vi "armff_arm_sim_init.vi"() -> (3 "SingleJointArmSim":T1 {"GearBox"."Jr_KgM2" format="%13.5p"; "GearBox"."L_H" format="%13.5p"; "GearBox"."Kt_NMPerAmp" format="%13.5p"; "GearBox"."KvINV_RadPerSecPerVolt" format="%13.5p"; "GearBox"."R_Ohms" format="%13.5p"; "GearBox"."FreeSpeed_RadPerSec" format="%13.5p"; "GearBox"."FreeCurrent_Amps" format="%13.5p"; "GearBox"."StallCurrent_Amps" format="%13.5p"; "GearBox"."StallTorque_NM" format="%13.5p"; "GearBox"."nominalVoltage_Volts" format="%13.5p"})   [LabVIEW 2019]
uses:
  <vilib>/Rock Robotics/WPI/ThirdParty/JAS_Junk/TrajLib/Trajectory_Library.lvlib
  <vilib>/Analysis/Matrix/Datatypes/RealMatrix.ctl
  <vilib>/Analysis/Matrix/NI_Matrix.lvlib
  <vilib>/Rock Robotics/WPI/ThirdParty/JAS_Junk/TrajLib/TypeDef/LINEAR_SYSTEM.ctl
  <vilib>/Rock Robotics/WPI/ThirdParty/JAS_Junk/TrajLib/TypeDef/LINEAR_SYSTEM_SIM.ctl
  <vilib>/Rock Robotics/WPI/ThirdParty/JAS_Junk/TrajLib/TypeDef/DCMOTOR.CTL
  <vilib>/Rock Robotics/WPI/ThirdParty/JAS_Junk/TrajLib/TypeDef/SINGLE_JOINT_ARM_SIM.ctl
panel:
  # "<States, 1>"
  # "<Outputs, 1>"
  # "<Inputs, 1>"
  # "<Outputs, 1>"
  # "<States,States>"
  # "<States,Inputs>"
  # "<Outputs,States>"
  # "<Outputs,Inputs>"
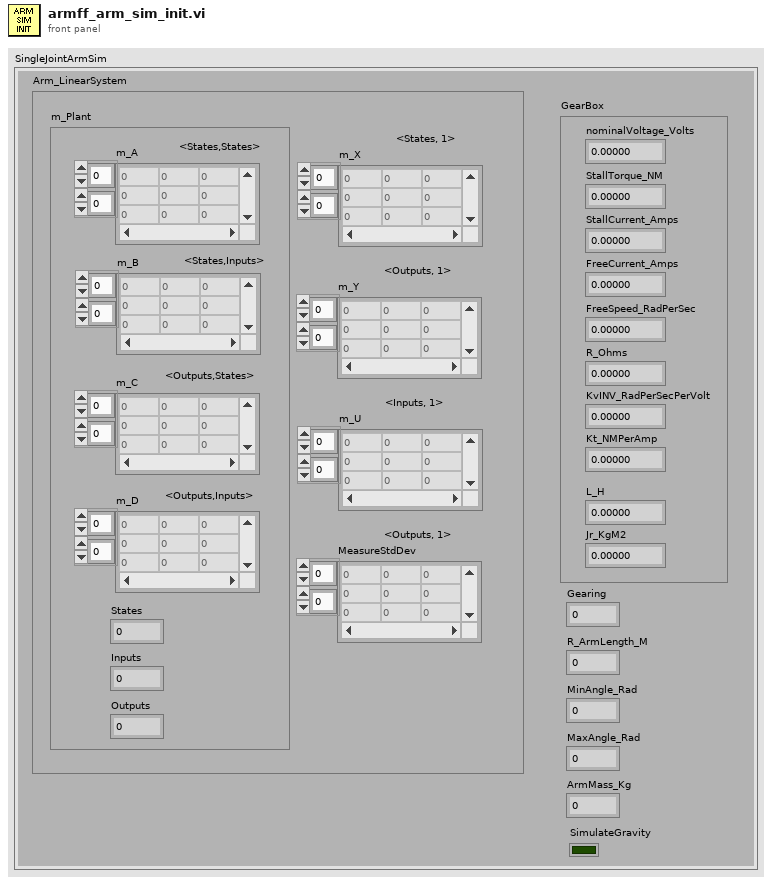
[diagram p1: front panel]
types:
  T1 = typedef "Trajectory_Library.lvlib/SINGLE_JOINT_ARM_SIM.ctl" = cluster{"Arm_LinearSystem":T2, "GearBox":T5, "Gearing":dbl, "R_ArmLength_M":dbl, "MinAngle_Rad":dbl, "MaxAngle_Rad":dbl, "ArmMass_Kg":dbl, "SimulateGravity":bool}
  T2 = typedef "Trajectory_Library.lvlib/LINEAR_SYSTEM_SIM.ctl" = cluster{"m_Plant":T3, "m_X":T4, "m_Y":T4, "m_U":T4, "MeasureStdDev":T4}
  T3 = typedef "Trajectory_Library.lvlib/LINEAR_SYSTEM.ctl" = cluster{"m_A":T4, "m_B":T4, "m_C":T4, "m_D":T4, "States":i32, "Inputs":i32, "Outputs":i32}
  T4 = typedef "NI_Matrix.lvlib/RealMatrix.ctl" = dbl[][]
  T5 = typedef "Trajectory_Library.lvlib/DCMOTOR.CTL" = cluster{"nominalVoltage_Volts":dbl, "StallTorque_NM":dbl, "StallCurrent_Amps":dbl, "FreeCurrent_Amps":dbl, "FreeSpeed_RadPerSec":dbl, "R_Ohms":dbl, "KvINV_RadPerSecPerVolt":dbl, "Kt_NMPerAmp":dbl, "L_H":dbl, "Jr_KgM2":dbl}
  T6 = typedef "Trajectory_Library.lvlib/KALMAN_FILTER.ctl" = cluster{"m_K":T4, "m_xHat":T4, "States":i32, "Outputs":i32, "m_Plant":T3}
  T7 = typedef "Trajectory_Library.lvlib/LINEAR_QUADRATIC_REGULATOR.ctl" = cluster{"m_r":T4, "m_U":T4, "m_K":T4, "States":i32, "Inputs":i32}
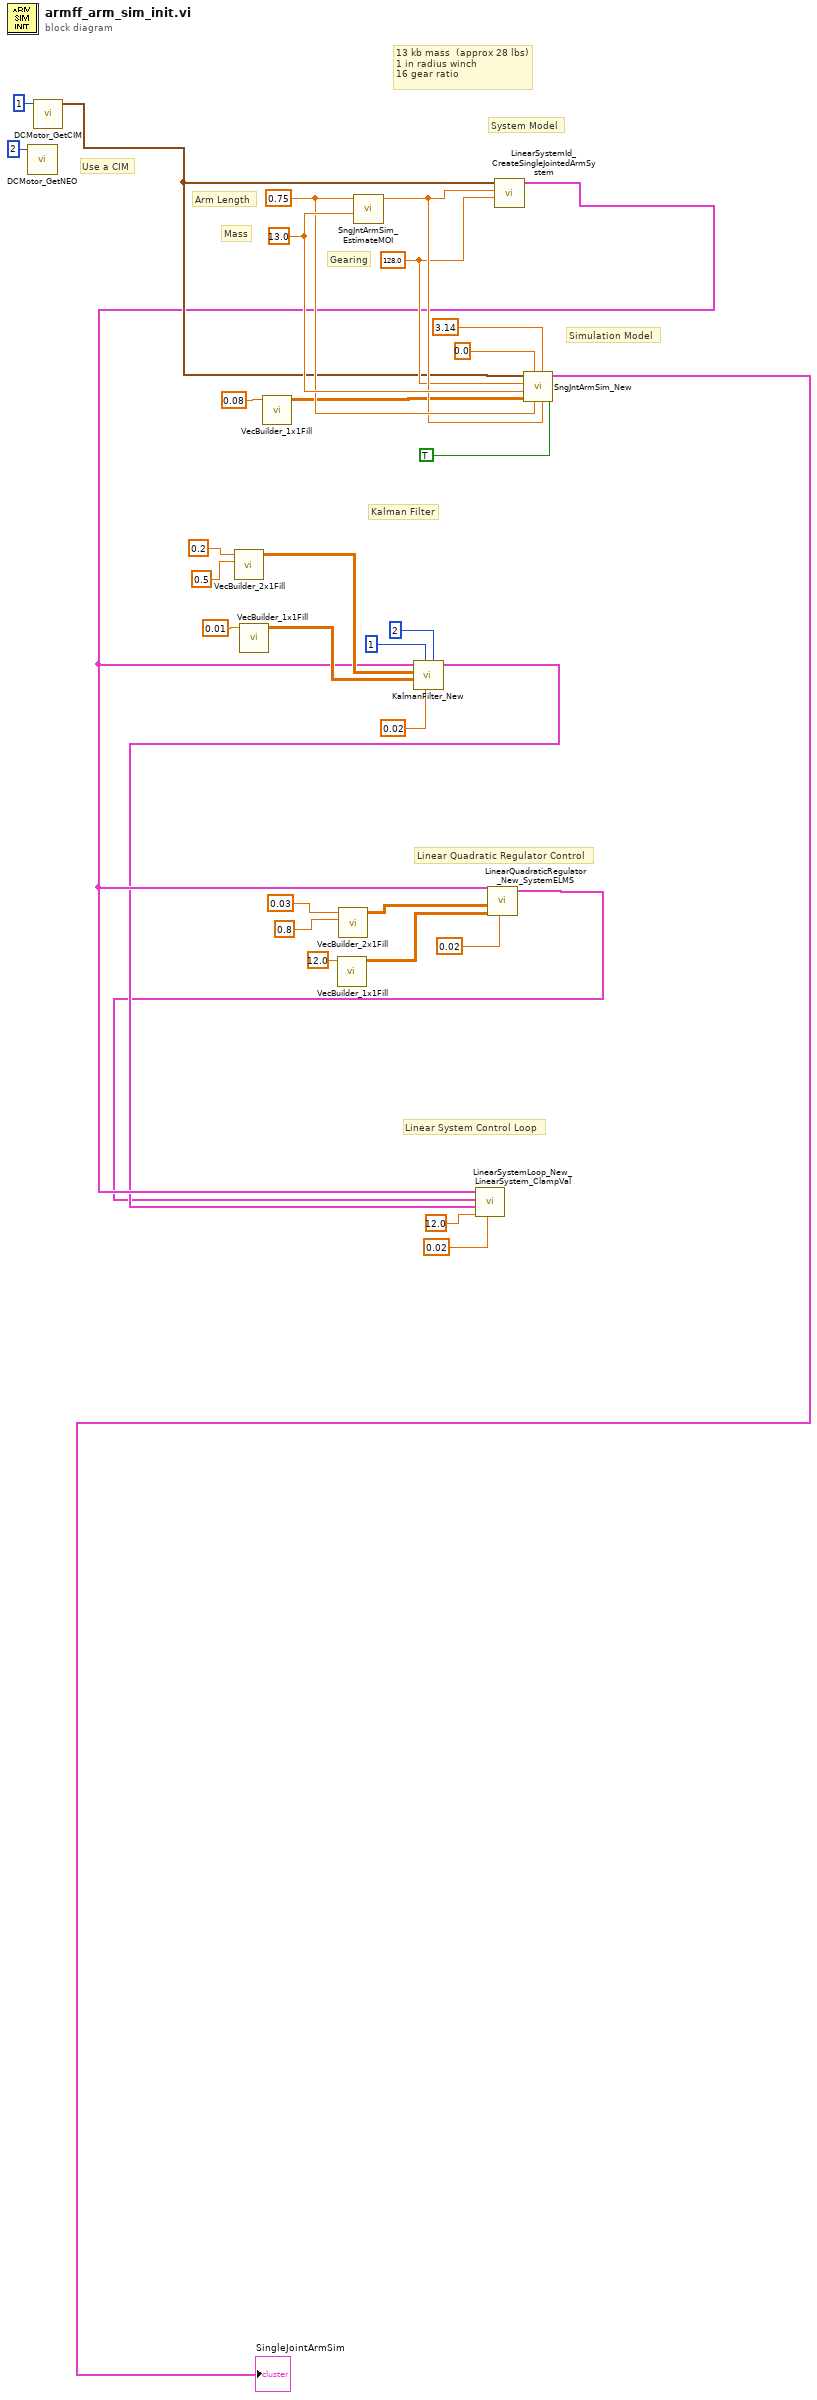
[diagram p0: block diagram]
diagram:
  w30 = 0.75 ("ArmLength_M")
  w27 = 128.0 ("G")
  w31 = 13.0 ("massKg")
  # "Simulation Model"
  # "System Model"
  # "Arm Length"
  # "Mass"
  # "Kalman Filter"
  # "Linear Quadratic Regulator Control"
  # "Linear System Control Loop"
  # "13 kb mass  (approx 28 lbs)\n1 in radius winch\n16 gear ratio"
  # "Gearing"
  # "Use a CIM"
  n1 = call <vilib>:"DCMotor_GetNEO.vi"("Num Motors"=2) -> ()  [unwired: 10 in, 1 out]
  n2 = call <vilib>:"DCMotor_GetCIM.vi"("Num Motors"=1) -> ("DCMOTOR"=w24:T5)  [unwired: 10 in]
  n3 = call <vilib>:"VecBuilder_2x1Fill.vi"("R1"=0.5, "R0"=0.2 ("R0_C0")) -> ("output matrix"=w12:T4)  [unwired: 9 in]
  n4 = call <vilib>:"VecBuilder_1x1Fill.vi"("R0_C0"=0.01) -> ("output matrix"=w13:T4)  [unwired: 10 in]
  n5 = call <vilib>:"VecBuilder_1x1Fill.vi"("R0_C0"=0.08) -> ("output matrix"=w28:T4)  [unwired: 10 in]
  n6 = call <vilib>:"VecBuilder_1x1Fill.vi"("R0_C0"=12.0) -> ("output matrix"=w19:T4)  [unwired: 10 in]
  n7 = call <vilib>:"VecBuilder_2x1Fill.vi"("R1"=0.8 ("R0_C0"), "R0"=0.03 ("R0_C0")) -> ("output matrix"=w17:T4)  [unwired: 9 in]
  n8 = call <vilib>:"SngJntArmSim_EstimateMOI.vi"("ArmMass_Kg"=w31, "ArmLength_M"=w30) -> ("MOI"=w29:dbl)  [unwired: 9 in]
  n9 = call <vilib>:"LinearSystemId_CreateSingleJointedArmSystem.vi"("G"=w27, "jKgSquaredMeters"=w29, "DCMOTOR"=w24) -> ("Linearsystem"=w6:T3)  [unwired: 7 in, 1 out]
  n10 = call <vilib>:"KalmanFilter_New.vi"("States"=2, "dt_Seconds"=0.02, "Outputs"=1, "MeasurementStdDevs"=w13, "StateStdDevs"=w12, "Plant"=w6) -> ("KalmanFilter"=w3:T6)  [unwired: 4 in, 1 out]
  n11 = call <vilib>:"LinearQuadraticRegulator_New_SystemELMS.vi"("dt_Seconds"=0.02, "Relms"=w19, "Qelms"=w17, "LINEARSYSTEM"=w6) -> ("LinearQuadraticRegulator"=w2:T7)  [unwired: 6 in, 1 out]
  n12 = call <vilib>:"LinearSystemLoop_New_LinearSystem_ClampVal.vi"("dT_Seconds"=0.02, "Max_Voltage"=12.0, "Observer"=w3, "Controller"=w2, "Plant"=w6) -> ()  [unwired: 5 in, 2 out]
  n13 = call <vilib>:"SngJntArmSim_New.vi"("SimulateGravity"=TRUE, "jKgMetersSquared"=w29, "MaxAngle_Rad"=3.14 ("MaxHeight_Meters"), "ArmLength_Meters"=w30, "MinAngle_Rad"=0.0 ("MinHeight_Meters"), "MeasurementStdDev"=w28, "ArmMass_Kg"=w31, "Gearing"=w27, "GearBox"=w24) -> ("SingleJointArmSim"=→"SingleJointArmSim":T1)  [unwired: 1 in, 1 out]
